vi "OAT Get Orbit Plot from Resampled Waveform.vi"(7 "tach duty":i32=1, 8 "trigger pulse direction":u16(ring)=1 items=["positive going", "negative going"], 9 "display revolutions":T1={"start (rev)"=0.0, "num of revolutions"=1.0} {"num of revolutions" format="%.2f"; "start (rev)" format="%.2f"}, 10 "resampled signal (Y)":cluster{"r0":dbl, "dr":dbl, "Y":dbl[]} {"r0" format="%.2p"; "dr" format="%.2p"; "Y" format="%.2f"}, 11 "resampled signal(X)":cluster{"r0":dbl, "dr":dbl, "Y":dbl[]} {"r0" format="%.2p"; "dr" format="%.2p"; "Y" format="%.2f"}) -> (3 "orbit plot data out":cluster{dbl[], dbl[]}[](array[cluster]) {"?" format="%.2f"; "?" format="%.2f"})   [LabVIEW 2017]
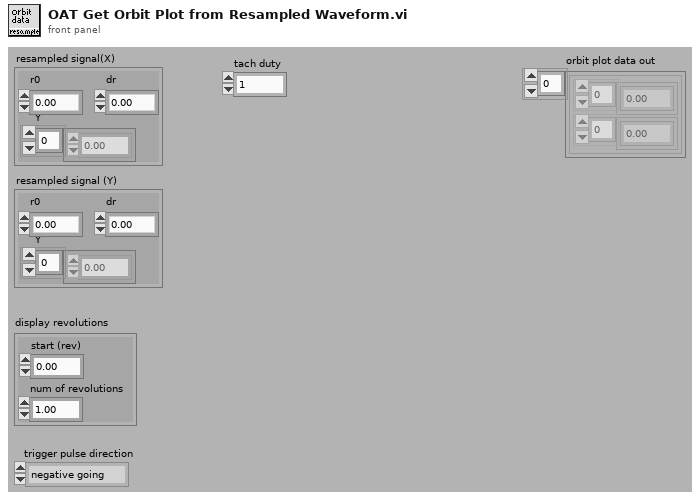
[diagram p1: front panel]
types:
  T1 = cluster{"start (rev)":dbl, "num of revolutions":dbl}
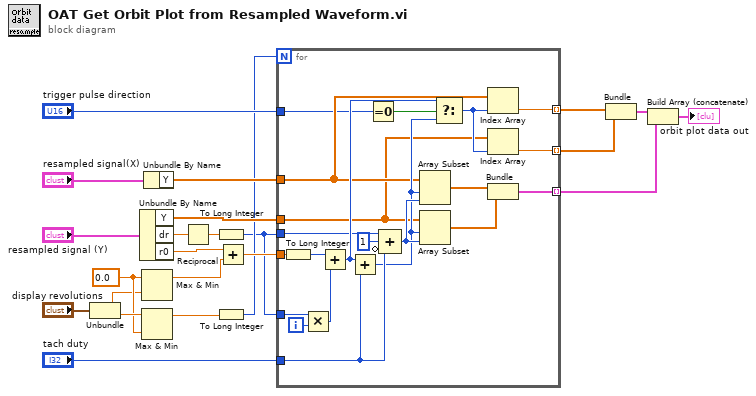
[diagram p0: block diagram]
diagram:
  w4 = 0.0 ("y")
  n1 = Unbundle("display revolutions") -> ("start (rev)"=w3:dbl, "num of revolutions"=w5:dbl)
  n2 = Unbundle By Name("resampled signal (Y)") -> ("Y"=w20:dbl[], "dr"=w8:dbl, "r0"=w18:dbl)
  n3 = Max & Min(x=w4, y=w3) -> (max(x,y)=w2:dbl)  [unwired: 1 out]
  n4 = Max & Min(x=w5, y=w4) -> (max(x,y)=w1:dbl)  [unwired: 1 out]
  n5 = Unbundle By Name("resampled signal(X)") -> ("Y"=w21:dbl[])
  n6 = Reciprocal(x=w8) -> (1/x=w7:dbl)
  n7 = To Long Integer(number=w7) -> (32bit integer=w6:i32)
  n8 = To Long Integer(number=w1) -> (32bit integer=w9:i32)
  n9 = Add(x=w18, y=w2) -> (x+y=w17:dbl)
  n10 = for {
    N: w9 -> [_]
    tunnel: w21 -> [w31]
    tunnel: w20 -> [w29]
    tunnel: w17 -> [w42]
    tunnel: "tach duty" -> [w39]
    tunnel: w6 -> [w24]
    tunnel: [w35] -> w11 mode=indexing
    tunnel: "trigger pulse direction" -> [w26]
    tunnel: [w28] -> w14 mode=indexing
    tunnel: [w27] -> w13 mode=indexing
    tunnel: w6 -> [w25]
    i -> [w44]
    n11 = To Long Integer(number=w42) -> (32bit integer=w41:i32)
    n12 = Multiply(x=w25, y=w44) -> (x*y=w43:i32)
    n13 = Add(x=w41, y=w43) -> (x+y=w33:i32)
    n14 = Add(x=w33, y=w39) -> (x+y=w32:i32)
    n15 = Equal To 0?(x=w26) -> (x = 0?=w34:bool)
    n16 = Compound Arithmetic op=unknown(w24, 1 ("value"), invert w39) -> (w38:i32)
    n17 = Array Subset(array=w31, index=w32, length=w38) -> (w37:dbl[])
    n18 = Array Subset(array=w29, index=w32, length=w38) -> (w36:dbl[])
    n19 = Select(t=w33, s=w34, f=w32) -> (s? t:f=w30:i32)
    n20 = Index Array(array=w31, index=w30) -> (element=w28:dbl)
    n21 = Index Array(array=w29, index=w30) -> (element=w27:dbl)
    n22 = Bundle(w37, w36) -> (w35:cluster{dbl[], dbl[]})  [unwired: 1 in]
  }
  n23 = Bundle(w14, w13) -> (w12:cluster{dbl[], dbl[]})  [unwired: 1 in]
  n24 = Build Array (concatenate)(w12, w11) -> (→"orbit plot data out":cluster{dbl[], dbl[]}[])
